vi "generateFilename.vi"(1 "Filename":string, 2 "Base path":path=path "C:/Users/sims01/Desktop/dataAcq") -> (0 "Appended path":path=path "C:/Users/LSFM_2/Desktop/dataAcq_2705/bothIllAxis/4umBead0.tif")   [LabVIEW 2015]
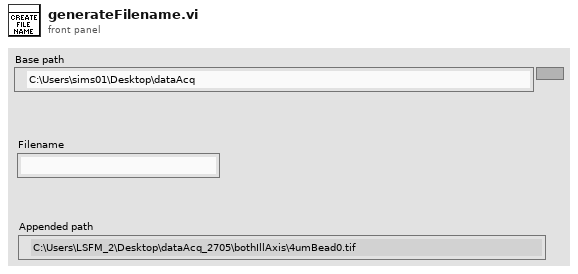
[diagram p1: front panel]
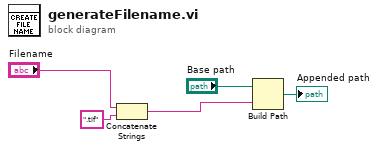
[diagram p0: block diagram]
diagram:
  n1 = Concatenate Strings("Filename", ".tif" ("string")) -> (w5:string)
  n2 = Build Path(base path="Base path", name or relative path=w5) -> (appended path=→"Appended path":path)
